vi "Fetch Part ID.vi"(11 "String":string) -> (3 "String 2":string)   [LabVIEW 2021]
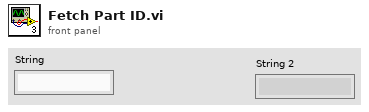
[diagram p1: front panel]
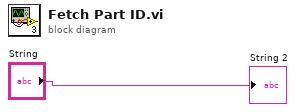
[diagram p0: block diagram]
diagram:
  "String 2" <- "String"
